vi "Parse EST Clusters into EST IP.vi"(8 "error in (no error)":errorcluster, 10 "EST version enum":T2, 11 "EPS IP LUT":variant) -> (0 "error out":errorcluster, 2 "Properties":T1[](array[typedef]), 3 "APUs":string[](array[string]))   [LabVIEW 2015, in "Engine Simulation Toolkit System Explorer.lvlib"]
uses:
  Engine Simulation Toolkit System Explorer.lvlib
  Shared/Bitfile EST Version.ctl
  String Array Property.ctl
  Shared/Properties.vi
  Shared/Engine Simulation Toolkit Shared.lvlib
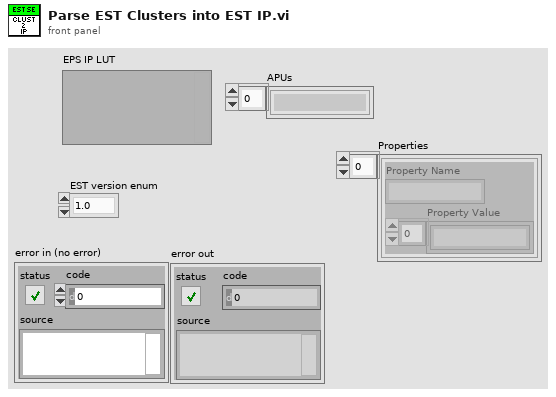
[diagram p1: front panel]
types:
  T1 = typedef "Engine Simulation Toolkit System Explorer.lvlib/String Array Property.ctl" = cluster{"Property Name":string, "Property Value":string[]}
  T2 = typedef "Engine Simulation Toolkit Shared.lvlib/Bitfile EST Version.ctl" = enum16{"1.0", "1.1", "1.2", "1.3"}
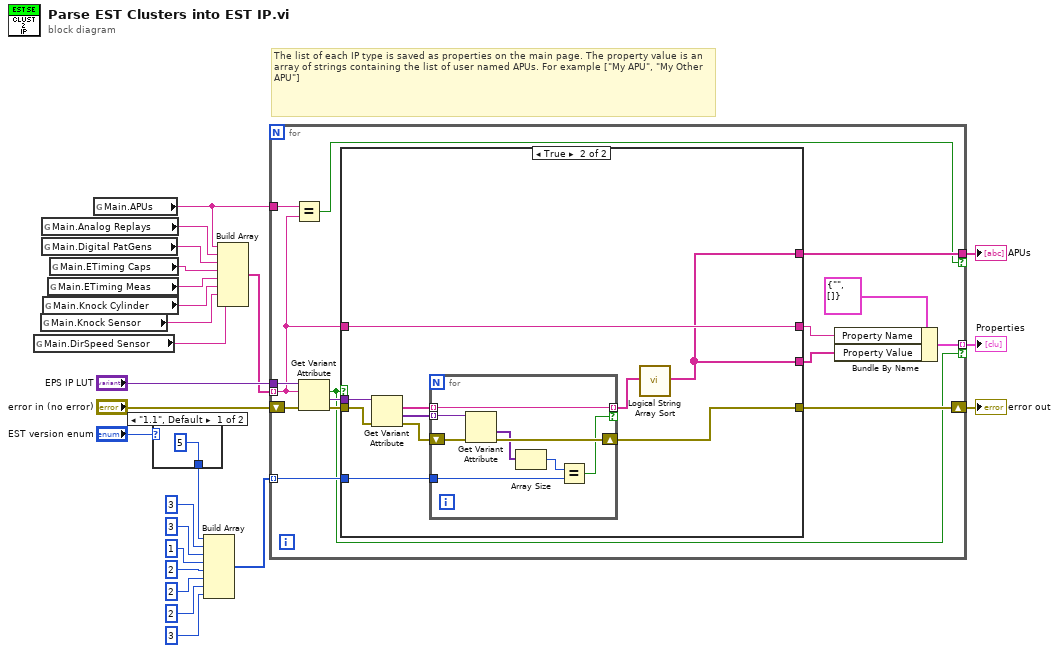
[diagram p0: block diagram]
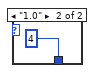
[diagram p2: hidden frame]
diagram:
  # "The list of each IP type is saved as properties on the main page. The property value is an array of strings containing the list of user named APUs. For example [\"My APU\", \"My Other APU\"]"
  n1 = global read "Properties.vi" "Main.DirSpeed Sensor"() -> (w4:string)
  n2 = global read "Properties.vi" "Main.Knock Sensor"() -> (w7:string)
  n3 = global read "Properties.vi" "Main.Analog Replays"() -> (w18:string)
  n4 = global read "Properties.vi" "Main.Digital PatGens"() -> (w17:string)
  n5 = global read "Properties.vi" "Main.Knock Cylinder"() -> (w8:string)
  n6 = global read "Properties.vi" "Main.ETiming Meas"() -> (w15:string)
  n7 = global read "Properties.vi" "Main.ETiming Caps"() -> (w16:string)
  n8 = global read "Properties.vi" "Main.APUs"() -> (w10:string)
  n9 = case shown="\"1.1\", Default" "EST version enum" {
    tunnel: [5 4] -> w19
    frame "1.1", Default {
    }
    frame "1.0" {
    }
  }
  n10 = Build Array(w19, 3, 3, 1, 2, 2, 2, 3) -> (w12:i32[])
  n11 = Build Array(w10, w18, w17, w16, w15, w8, w7, w4) -> (w13:string[])
  n12 = for {
    shift-right: [w37] -> w11
    shift-left: "error in (no error)" -> [w41]
    tunnel: "EPS IP LUT" -> [w40]
    tunnel: w13 -> [w35] mode=indexing
    tunnel: w12 -> [w36] mode=indexing
    tunnel: w10 -> [w34]
    tunnel: [w33] -> w9 if=w32
    tunnel: [w29] -> w1 mode=indexing if=w28
    n13 = Equal?(x=w34, y=w35) -> (x = y?=w32:bool)
    n14 = Get Variant Attribute(Variant=w40, name=w35, error in=w41) -> (found=w28:bool, value=w38:variant, error out=w39:errorcluster)  [unwired: 1 in, 1 out]
    n15 = case shown="True" w28 {
      tunnel: w39 -> [w43 w52]
      tunnel: w38 -> [_ w53]
      tunnel: [w43 w44] -> w37
      tunnel: w36 -> [_ w51]
      tunnel: w35 -> [w42 w46]
      tunnel: [_ w45] -> w33
      tunnel: [w42 w46] -> w31
      tunnel: [_ w45] -> w30
      frame False {
      }
      frame True {
        n16 = Get Variant Attribute(Variant=w53, error in=w52) -> (names=w49:string[], values=w48:variant[], error out=w50:errorcluster)  [unwired: 2 in, 1 out]
        n17 = for {
          tunnel: w51 -> [w61]
          shift-right: [w57] -> w44
          shift-left: w50 -> [w58]
          tunnel: w49 -> [w55] mode=indexing
          tunnel: w48 -> [w59] mode=indexing
          tunnel: [w55] -> w47 mode=indexing if=w54
          n18 = Get Variant Attribute(Variant=w59, error in=w58) -> (values=w56:variant[], error out=w57:errorcluster)  [unwired: 2 in, 2 out]
          n19 = Array Size(array=w56) -> (size(s)=w60:i32)
          n20 = Equal?(x=w60, y=w61) -> (x = y?=w54:bool)
        }
        n21 = call "Logical String Array Sort.vi"("Unsorted List"=w47) -> ("Sorted List"=w45:string[])  [unwired: 18 in]
      }
    }
    n22 = Bundle By Name(cluster=T1 {"Property Name"="", "Property Value"=[]} ("String Array Property"), "Property Name"=w31, "Property Value"=w30) -> (w29:T1)
  }
  "error out" <- w11
  "APUs" <- w9
  "Properties" <- w1
